vi "LWXPS_GlobalArrayGet.vi"(0 "XPS Reference IN":refnum<k24>, 5 "Number":i32, 11 "LabVIEW error IN":errorcluster) -> (4 "XPS Reference OUT":refnum<k24>, 6 "Returned error code":i32, 8 "Value String":string, 10 "XPS Error String":string, 15 "LabVIEW error OUT":errorcluster)   [LabVIEW 2014]
uses:
  D:/XPSQ8_LabView_Library/Development/Source/Dll/Newport.XPS.CommandInterface.dll
  Dll/Newport.XPS.CommandInterface.dll
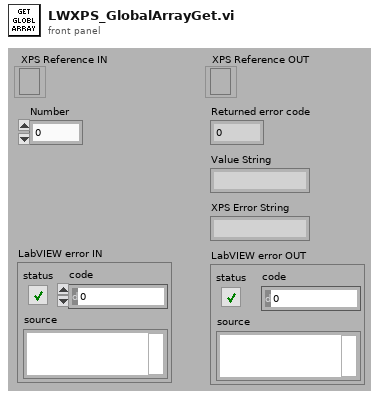
[diagram p1: front panel]
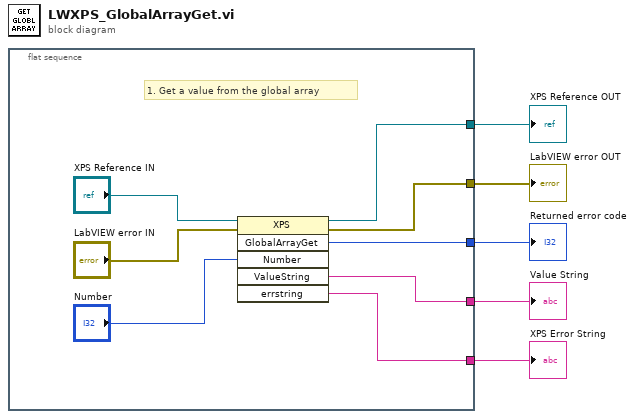
[diagram p0: block diagram]
diagram:
  n1 = flat-sequence {
    tunnel: [w8] -> w5
    tunnel: [w12] -> w4
    tunnel: [w10] -> w3
    tunnel: [w9] -> w2
    tunnel: [w7] -> w1
    frame #0 {
      # "1. Get a value from the global array"
      n2 = invoke class="XPS" method="GlobalArrayGet"(reference="XPS Reference IN", error in="LabVIEW error IN", "Number"="Number") -> (reference out=w8:refnum<k24>, error out=w12:errorcluster, "GlobalArrayGet"=w10:i32, "ValueString"=w9:string, "errstring"=w7:string)  [unwired: 3 in, 1 out]
    }
  }
  "XPS Reference OUT" <- w5
  "LabVIEW error OUT" <- w4
  "Returned error code" <- w3
  "XPS Error String" <- w1
  "Value String" <- w2
